vi "OS_Var_to_Comm_Analog.vi"() -> (1 "Array":dbl[](array[numeric]), 2 "Array 2":u16[](array[numeric]))   [LabVIEW 2016, in "DNP3_Outstation_Template.lvlib"]
uses:
  DNP3_Outstation_Template.lvlib
  <vilib>/Utility/file.llb/Read Delimited Spreadsheet (string).vi
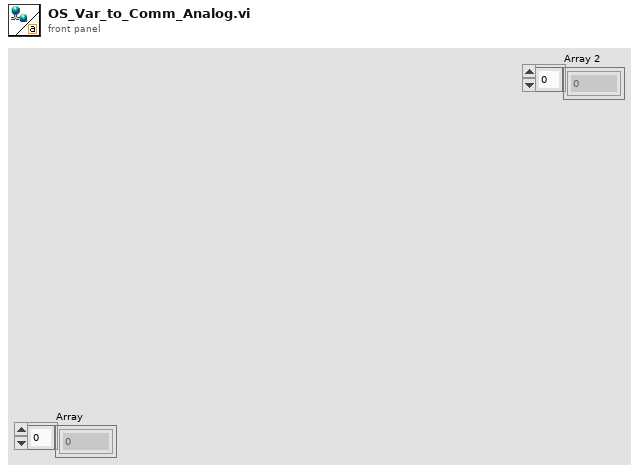
[diagram p1: front panel]
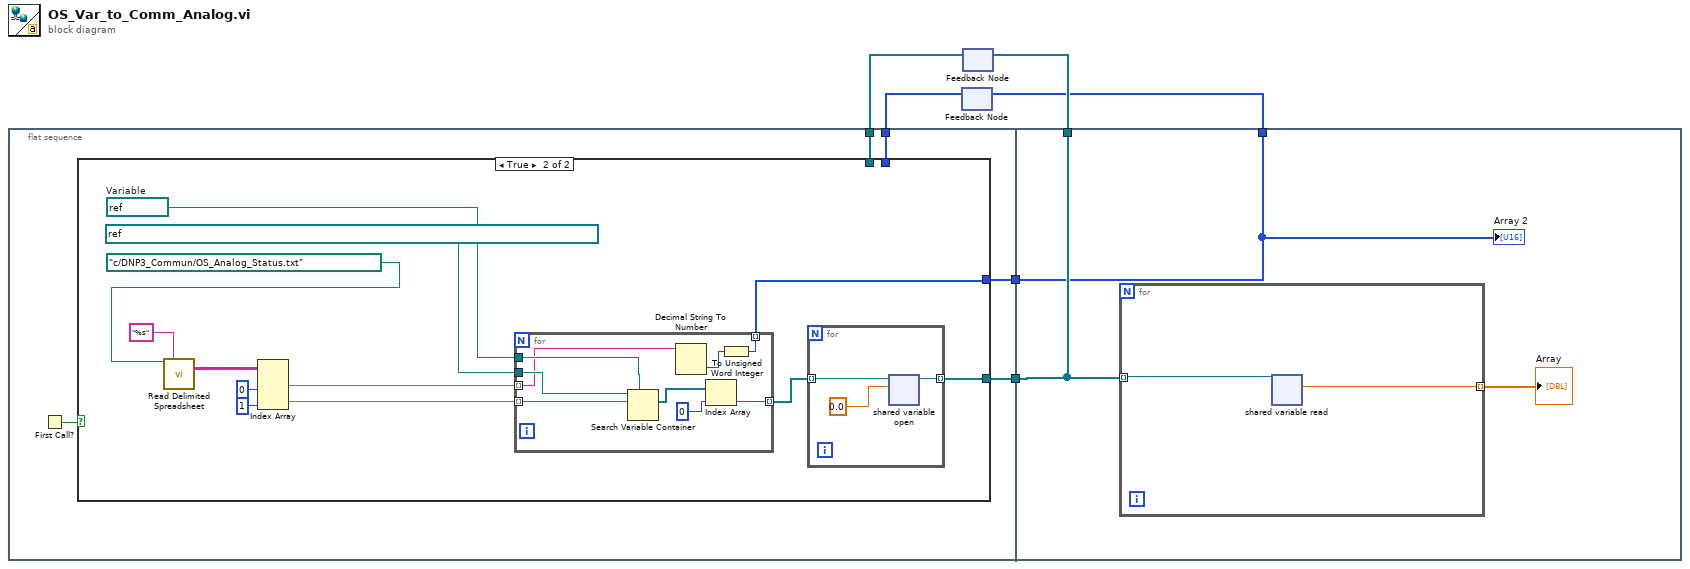
[diagram p0: block diagram]
diagram:
  n1 = flat-sequence {
    tunnel: [w10] -> w6
    tunnel: w4 -> [w9]
    tunnel: [w8] -> w3
    tunnel: w1 -> [w7]
    tunnel: w6 -> [w39]
    tunnel: [w39] -> w5
    tunnel: w3 -> [w38]
    tunnel: [w38] -> w2
    frame #0 {
      n2 = First Call?() -> (First Call?: T/F=w11:bool)
      n3 = case shown="True" w11 {
        tunnel: [w13 w15] -> w10
        tunnel: w9 -> [w13 _]
        tunnel: [w12 w14] -> w8
        tunnel: w7 -> [w12 _]
        frame False {
        }
        frame True {
          w17 = refnum<k21> refnum  # Variable
          n4 = call-poly <vilib>:"Read Delimited Spreadsheet.vi"("file path (dialog if empty)"=path "c:/DNP3_Commun/OS_Analog_Status.txt" ("file path (use dialog)"), "format (%s)"="%s") -> ("all rows"=w21:string[][])  [unwired: 8 in, 5 out]
          n5 = Index Array(array=w21, index (col) #1=0 ("disabled index (col)"), index (col) #2=1 ("index (col)")) -> (element #1=w24:string[], element #2=w25:string[])  [unwired: 2 in]
          n6 = for {
            tunnel: w17 -> [w35]
            tunnel: refnum<k21> "ni.var.psp://lc1 (bess)/DNP3_Outstation_Template/OS_Data_Variables/OS_Analog_Status" ("container refnum in") -> [w34]
            tunnel: w24 -> [w31] mode=indexing
            tunnel: w25 -> [w33] mode=indexing
            tunnel: [w32] -> w16 mode=indexing
            tunnel: [w30] -> w14 mode=indexing
            n7 = Search Variable Container(7:w35, 10:w33, 11:w34) -> (2:w37:refnum<k21>[])  [unwired: 3 in, 2 out]
            n8 = Decimal String To Number(string=w31) -> (number=w29:i32)  [unwired: 2 in, 1 out]
            n9 = Index Array(array=w37, index=0) -> (element=w32:refnum<k21>)
            n10 = To Unsigned Word Integer(number=w29) -> (unsigned 16bit integer=w30:u16)
          }
          n11 = for {
            tunnel: w16 -> [w27] mode=indexing
            tunnel: [w26] -> w15 mode=indexing
            n12 = shared-variable-open(w27, 0.0) -> (w26:refnum<k21>)  [unwired: 2 in, 1 out]
          }
        }
      }
    }
    frame #1 {
      n13 = for {
        tunnel: w39 -> [w41] mode=indexing
        tunnel: [w42] -> w40 mode=indexing
        n14 = shared-variable-read(w41) -> (w42:dbl)  [unwired: 1 in, 3 out]
      }
      "Array" <- w40
      "Array 2" <- w38
    }
  }
  n15 = feedback #1() -> (w1:u16[])  [unwired: 1 in]
  n16 = feedback-in #1(w2) -> ()
  n17 = feedback-in #2(w5) -> ()
  n18 = feedback #2() -> (w4:refnum<k21>[])  [unwired: 1 in]
